vi "HandShaking.vi"(6 "Elapsed Time":u32, 8 "error in":errorcluster, 10 "Event Sources":T1, 11 "Ignition in":refnum<class "Ignition.lvclass">) -> (0 "error out":errorcluster, 3 "Ignition out":refnum<class "Ignition.lvclass">)   [LabVIEW 2021, in "OPC UA.lvlib" / "Ignition.lvclass"]
uses:
  Ignition.lvclass
  Ignition.lvclass/Ignition.ctl
  <vilib>/addons/TestStand/_TSUtility.llb/TestStand - Get Property Value (String).vi
  OPC UA/OPC UA.lvclass
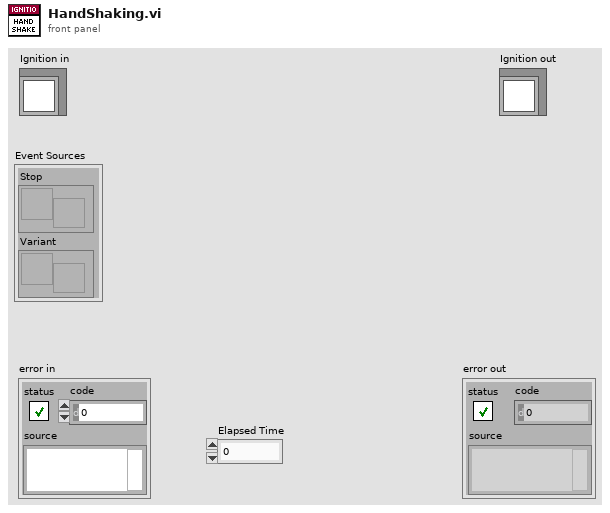
[diagram p1: front panel]
types:
  T1 = cluster{"Stop":refnum<user-event>, "Variant":refnum<user-event>}
  T2 = typedef "Ignition.lvclass/Tester Rx.ctl" = cluster{"result_ack":bool}
  T3 = typedef "Ignition.lvclass/Tester Tx.ctl" = cluster{"thermistor":dbl, "phase_angle":dbl, "pallet_rfid":dbl, "ocv":dbl, "cell_vsense1":dbl, "cell_vsense2":dbl, "hipot1_leakage_current":dbl, "hipot2_leakage_current":dbl, "guid":string, "can_sn":string, "can_pn":string, "ac_internal_resistance":dbl, "sub_station":string, "fault_code":i32, "elapsed_time":i32, "result":i32, "reject_code_reason":string, "result_ready":bool, "Timeout":bool}
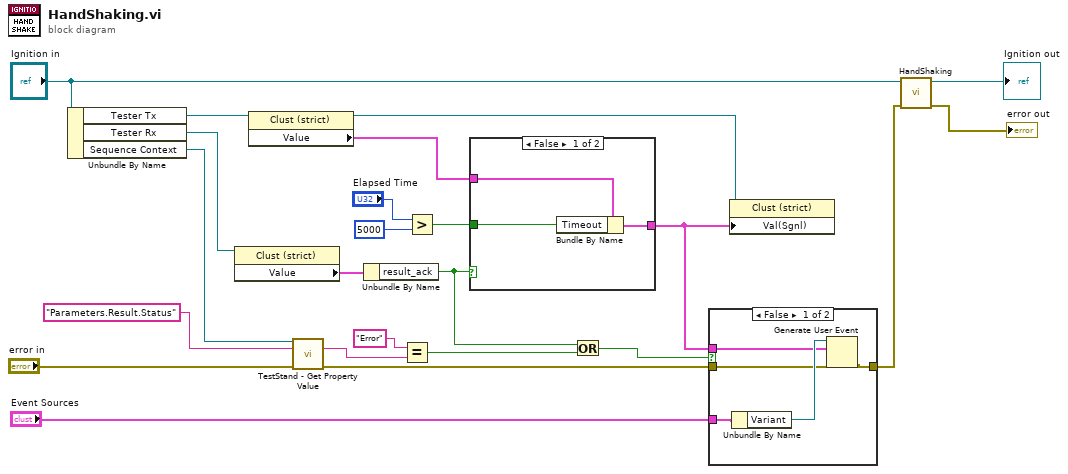
[diagram p0: block diagram]
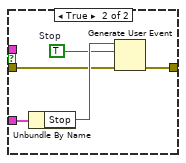
[diagram p2: hidden frame]
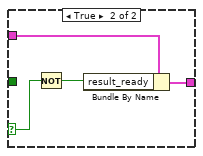
[diagram p3: hidden frame]
diagram:
  n1 = Unbundle By Name("Ignition in") -> ("Tester Tx"=w20:refnum<vi>, "Tester Rx"=w15:refnum<vi>, "Sequence Context"=w8:refnum<k7>)
  n2 = property class="Clust (strict)"(reference=w15) -> ("Value"=w14:T2)  [unwired: 1 in, 2 out]
  n3 = property class="Clust (strict)"(reference=w20) -> (reference out=w19:refnum<vi>, "Value"=w2:T3)  [unwired: 1 in, 1 out]
  n4 = call-poly <vilib>:"TestStand - Get Property Value.vi"("Sequence Context In"=w8, "Lookup String"="Parameters.Result.Status", "error in (no error)"="error in") -> ("Value"=w9:string, "error out"=w5:errorcluster)  [unwired: 10 in, 1 out]
  n5 = Unbundle By Name(w14) -> ("result_ack"=w1:bool)
  n6 = Equal?(x="Error" ("Lookup String"), y=w9) -> (x = y?=w4:bool)
  n7 = Greater?(x="Elapsed Time", y=u32 5000) -> (0:w16:bool)
  n8 = case shown="False" w1 {
    selector: w1 -> [_ w28]
    tunnel: w2 -> [w26 w30]
    tunnel: [w25 w29] -> w13
    tunnel: w16 -> [w24 _]
    frame False {
      n9 = Bundle By Name(cluster=w26, "Timeout"=w24) -> (w25:T3)
    }
    frame True {
      n10 = Not(x=w28) -> (.not. x?=w27:bool)
      n11 = Bundle By Name(cluster=w30, "result_ready"=w27) -> (w29:T3)
    }
  }
  n12 = Or(x=w1, y=w4) -> (x .or. y?=w3:bool)
  n13 = case shown="False" w3 {
    tunnel: "Event Sources" -> [w35 w40]
    tunnel: w13 -> [w33 _]
    tunnel: w5 -> [w32 w37]
    tunnel: [w31 w36] -> w11
    frame False {
      n14 = Unbundle By Name(w35) -> ("Variant"=w34:refnum<user-event>)
      n15 = Generate User Event(user event=w34, event data cluster=w33, error in=w32) -> (error out=w31:errorcluster)  [unwired: 1 in, 1 out]
    }
    frame True {
      w38 = TRUE  # Stop
      n16 = Unbundle By Name(w40) -> ("Stop"=w39:refnum<user-event>)
      n17 = Generate User Event(user event=w39, event data cluster=w38, error in=w37) -> (error out=w36:errorcluster)  [unwired: 1 in, 1 out]
    }
  }
  n18 = property class="Clust (strict)"(reference=w19, "Val(Sgnl)"=w13) -> ()  [unwired: 1 in, 2 out]
  n19 = call-parent "HandShaking.vi"("error in (no error)"=w11, "OPC UA in"="Ignition in") -> ("error out"=→"error out":errorcluster, "OPC UA out"=→"Ignition out":refnum<class "Ignition.lvclass">)  [unwired: 8 in]
